vi "Xctrl interface-Set trial cursors.vi"(8 "error in (no error)":errorcluster) -> (0 "error out":errorcluster)   [LabVIEW 2020]
uses:
  XGrapher.xctl
  Global variables/gl_Functional Imaging-Global variables.vi
panel:
  out "POI data points in each trial":i32
  out "Trial number":i32
  out "Trial duration (s)":dbl
  out "Cursor positions":cluster{"Left":dbl, "Right":dbl}
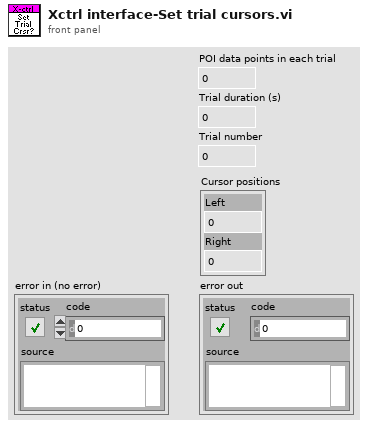
[diagram p1: front panel]
types:
  T1 = typedef "Functional Imging UI Refs.ctl" = cluster{"Menu ref":refnum<k9>, "Image control":refnum<vi>, "VI ref":refnum<vi>, "XGrapher":refnum<vi>, "Smoothing":refnum<vi>, "POI Averaging":refnum<vi>, "Normalize":refnum<vi>, "POI data points in each trial":refnum<vi>, "Channel":refnum<vi>, "Experiment data folder path":refnum<vi>, "[ROI vis]":refnum<vi>, "[Groups] visbl":T2, "Group Name":refnum<vi>, "POI index":refnum<vi>, "Trial No.":refnum<vi>, "Intensity Zoom":refnum<vi>, "Trial Cursor Enabled":refnum<vi>, "Number of Trials (ind 1)":refnum<vi>, "Number of Trials (ind 2)":refnum<vi>, "MiniScans Available":refnum<vi>, "POI Available":refnum<vi>, "Defer graph updates":refnum<vi>, "Waveform selector":refnum<vi>, "#of selected POI":refnum<vi>, "#of selected MiniScans":refnum<vi>, "#of selected groups":refnum<vi>, "Max Z-Projection":refnum<vi>, "Z-Plane Selector":refnum<vi>, "Index of miniscan point to visualise":refnum<vi>, "ROI vis. mode":refnum<vi>, "Total # of points":refnum<vi>, "Index of group clicked on":refnum<vi>, "Pane 1":refnum<vi>, "Pane 2":refnum<vi>, "Pane 3":refnum<vi>, "Pane 4":refnum<vi>, "Pane 5":refnum<vi>, "Pane 6":refnum<vi>, "Deselect all ROI":refnum<vi>, "Deselect all groups":refnum<vi>}
  T2 = typedef "Groups array referecne.ctl" = refnum<vi>
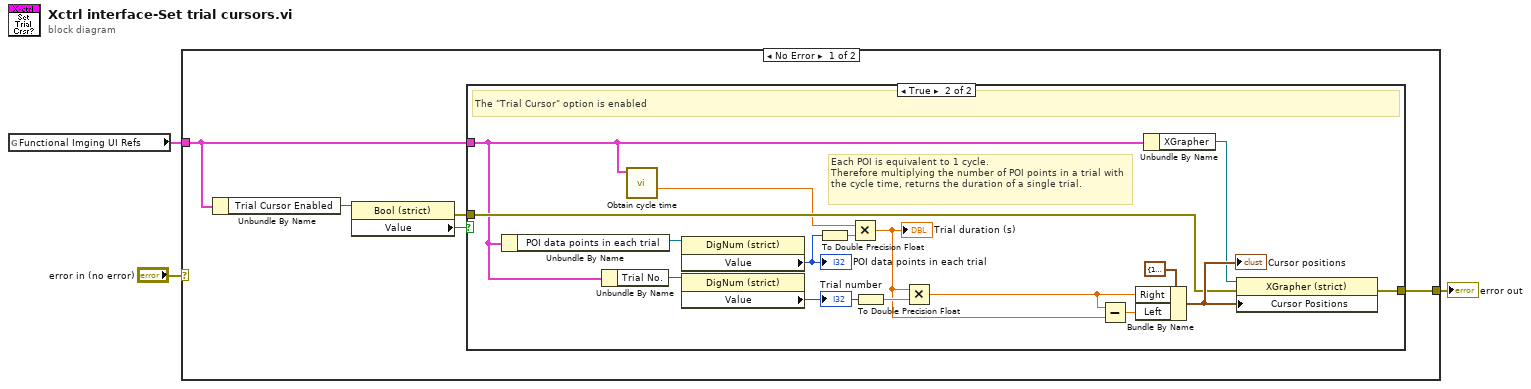
[diagram p0: block diagram]
diagram:
  n1 = global read "gl_Functional Imaging-Global variables.vi" "Functional Imging UI Refs"() -> (w1:T1)
  n2 = case shown="No Error" "error in (no error)" {
    selector: "error in (no error)" -> [_ w26]
    tunnel: [w8 w26] -> w3
    tunnel: w1 -> [w7 _]
    frame No Error {
      n3 = Unbundle By Name(w7) -> ("Trial Cursor Enabled"=w6:refnum<vi>)
      n4 = property on="Property Node" class="Bool (strict)"(reference=w6) -> (error out=w4:errorcluster, "Value"=w5:bool)  [unwired: 1 in, 1 out]
      n5 = case shown="True" w5 {
        tunnel: [w9 w25] -> w8
        tunnel: w7 -> [_ w11]
        tunnel: w4 -> [w9 w13]
        frame False {
          # "The \"Trial Cursor\" option is disabled"
        }
        frame True {
          # "Each POI is equivalent to 1 cycle.\nTherefore multiplying the number of POI points in a trial with the cycle time, returns the duration of a single trial."
          # "The \"Trial Cursor\" option is enabled"
          n6 = Unbundle By Name(w11) -> ("POI data points in each trial"=w23:refnum<vi>)
          n7 = Unbundle By Name(w11) -> ("Trial No."=w21:refnum<vi>)
          n8 = call "Obtain cycle time.vi"("Functional Imging UI Refs"=w11) -> ("Funct Acq Cycle time (sec)"=w10:dbl)  [unwired: 6 in, 4 out]
          n9 = property on="Property Node" class="DigNum (strict)"(reference=w23) -> ("Value"=w24:i32)  [unwired: 1 in, 2 out]
          "POI data points in each trial" <- w24
          n10 = property on="Property Node" class="DigNum (strict)"(reference=w21) -> ("Value"=w22:i32)  [unwired: 1 in, 2 out]
          "Trial number" <- w22
          n11 = To Double Precision Float(number=w24) -> (double precision float=w18:dbl)
          n12 = Multiply(x=w10, y=w18) -> (x*y=w15:dbl)
          "Trial duration (s)" <- w15
          n13 = To Double Precision Float(number=w22) -> (double precision float=w19:dbl)
          n14 = Multiply(x=w15, y=w19) -> (x*y=w14:dbl)
          n15 = Subtract(x=w14, y=w15) -> (x-y=w16:dbl)
          n16 = Bundle By Name(cluster=cluster{"Left":dbl, "Right":dbl} {"Left"=10.0, "Right"=90.0} ("Cursor Positions"), "Right"=w14, "Left"=w16) -> (w17:cluster{"Left":dbl, "Right":dbl})
          "Cursor positions" <- w17
          n17 = Unbundle By Name(w11) -> ("XGrapher"=w12:refnum<vi>)
          n18 = property on="Property Node" class="XGrapher (strict)"(reference=w12, error in=w13, "Cursor Positions"=w17) -> (error out=w25:errorcluster)  [unwired: 1 out]
        }
      }
    }
    frame Error {
    }
  }
  "error out" <- w3
